vi "CONEX - Wait for MOVE complete.vi"(7 "Timeout (ms)":dbl=10000.0 format="%#_13g", 11 "Connection Cluster in":T1) -> (2 "Timout Error":bool, 3 "Connection Cluster out":T1)   [LabVIEW 2014]
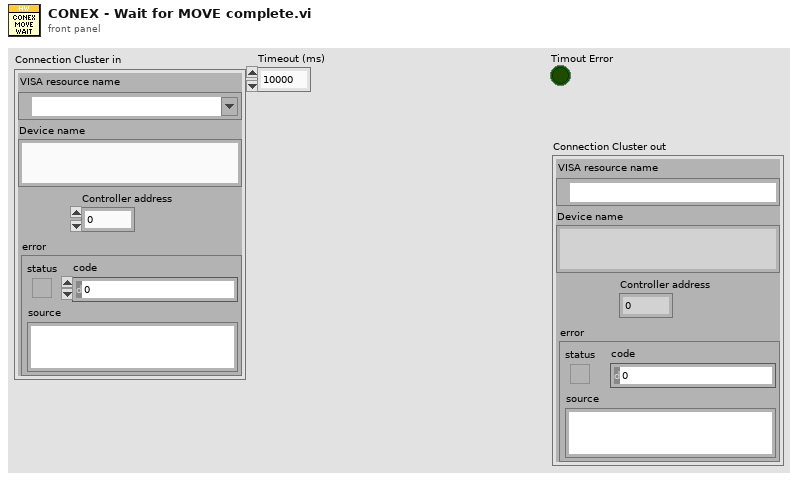
[diagram p1: front panel]
types:
  T1 = cluster{"VISA resource name":refnum<visa-resource-name>, "Device name":string, "Controller address":i32, "error":errorcluster}
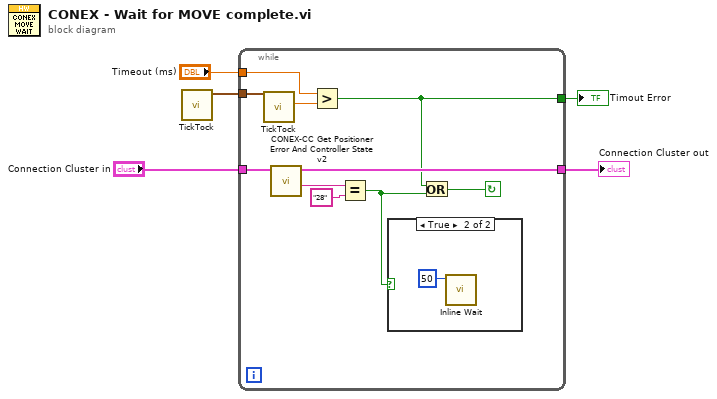
[diagram p0: block diagram]
diagram:
  n1 = call "TickTock.vi"() -> ("Current Time (Out)"=w3:timestamp)  [unwired: 9 in, 2 out]
  n2 = while {
    tunnel: "Connection Cluster in" -> [w15]
    tunnel: [w12] -> w4
    tunnel: w3 -> [w10]
    tunnel: "Timeout (ms)" -> [w8]
    tunnel: [w6] -> w1
    stop <- w7 continue-if-true
    n3 = call "TickTock.vi"("Current Time (In)"=w10) -> ("dt"=w9:dbl)  [unwired: 8 in, 2 out]
    n4 = call "CONEX-CC Get Positioner Error And Controller State v2.vi"("Connection Cluster in"=w15) -> ("Controller state"=w13:string, "Connection Cluster out"=w12:T1)  [unwired: 8 in, 1 out]
    n5 = Greater?(x=w8, y=w9) -> (0:w6:bool)
    n6 = Equal?(x=w13, y="28") -> (x = y?=w11:bool)
    n7 = case shown="True" w11 {
      frame False {
      }
      frame True {
        n8 = call "Inline Wait.vi"("milliseconds to wait"=u32 50) -> ()  [unwired: 10 in, 1 out]
      }
    }
    n9 = Or(x=w6, y=w11) -> (x .or. y?=w7:bool)
  }
  "Connection Cluster out" <- w4
  "Timout Error" <- w1
